vi "DB_Lee_IP_ID_NOMBE_equipos.vi"() -> (0 "error out":errorcluster, 1 "NOMBRE_EQUIPOS":string[](array[string]), 2 "IP_EQUIPO":string[](array[string]), 3 "ID_EQUIPO":i32[](array[numeric]))   [LabVIEW 2018]
uses:
  <vilib>/addons/database/Connection.llb/DB Tools Open Connec (Path).vi
  <vilib>/addons/database/Connection.llb/Conn Execute.vi
  <vilib>/addons/database/Recordset.llb/Rec Fetch Recordset Data (R).vi
  <vilib>/addons/database/Recordset.llb/Rec Destroy - Connection.vi
  <vilib>/addons/database/_DB Variant To Data/Database Variant To Data.xnode
  <vilib>/addons/database/NI_Database_API.lvlib
panel:
  in  "error in (no error)":errorcluster
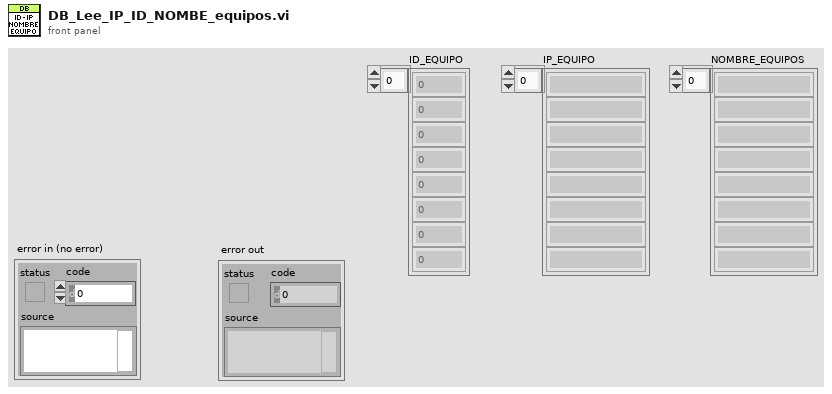
[diagram p1: front panel]
types:
  T1 = typedef "NI_Database_API.lvlib/Conn ObjectReference.ctl" = refnum<k1>
  T2 = typedef "NI_Database_API.lvlib/Rec ObjectReference.ctl" = refnum<k1>
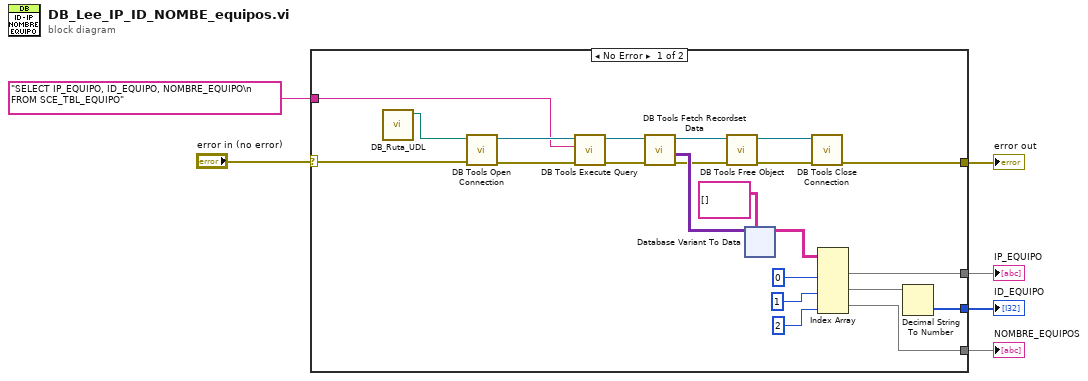
[diagram p0: block diagram]
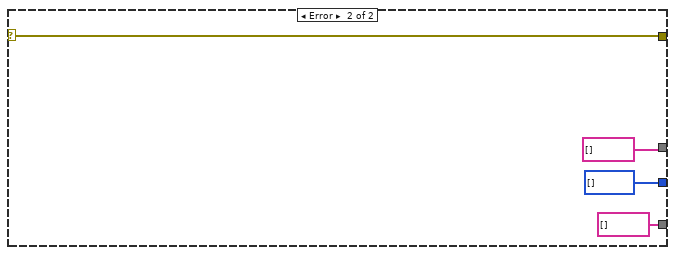
[diagram p2: hidden frame]
diagram:
  n1 = case shown="No Error" "error in (no error)" {
    selector: "error in (no error)" -> [w23 w76]
    tunnel: [w25 w76] -> w6
    tunnel: "SELECT IP_EQUIPO, ID_EQUIPO, NOMBRE_EQUIPO\n  FROM SCE_TBL_EQUIPO" ("SQL") -> [w22 _]
    tunnel: [w11 i32[] []] -> w3
    tunnel: [w13 string[] [] ("data")] -> w2
    tunnel: [w8 string[] [] ("data")] -> w1
    frame No Error {
      n2 = call "DB_Ruta_UDL.vi"() -> ("UDL ruta"=w10:path)  [unwired: 11 in]
      n3 = call-poly <vilib>:"DB Tools Open Connection.vi"("error in (no error)"=w23, "connection information"=w10) -> ("error out"=w28:errorcluster, "connection reference"=w26:T1)  [unwired: 6 in]
      n4 = call-poly <vilib>:"DB Tools Execute Query.vi"("error in (no error)"=w28, "SQL query"=w22, "connection reference"=w26) -> ("error out"=w24:errorcluster, "recordset reference"=w21:T2)  [unwired: 5 in]
      n5 = call-poly <vilib>:"DB Tools Fetch Recordset Data.vi"("error in (no error)"=w24, "recordset reference"=w21) -> ("error out"=w17:errorcluster, "recordset data"=w18:variant[][], "recordset reference out"=w20:T2)  [unwired: 3 in]
      n6 = call-poly <vilib>:"DB Tools Free Object.vi"("error in (no error)"=w17, "recordset reference"=w20) -> ("error out"=w27:errorcluster, "connection reference"=w7:T1)  [unwired: 8 in]
      n7 = xnode "Database Variant To Data"("database variant"=w18, "type"=string[][] []) -> ("data"=w16:string[][])  [unwired: 1 in, 1 out]
      n8 = call <vilib>:"DB Tools Close Connection.vi"("error in (no error)"=w27, "connection reference"=w7) -> ("error out"=w25:errorcluster)  [unwired: 5 in]
      n9 = Index Array(array=w16, index (col) #1=0 ("disabled index (col)"), index (col) #2=1 ("index (col)"), index (col) #3=2 ("index (col)")) -> (element #1=w13:string[], element #2=w12:string[], element #3=w8:string[])  [unwired: 3 in]
      n10 = Decimal String To Number(string=w12) -> (number=w11:i32[])  [unwired: 2 in, 1 out]
    }
    frame Error {
    }
  }
  "error out" <- w6
  "ID_EQUIPO" <- w3
  "IP_EQUIPO" <- w2
  "NOMBRE_EQUIPOS" <- w1
